vi "Set IConfiguration.vi"(8 "error in":errorcluster, 10 "IConfiguration":refnum<class "IConfiguration.lvclass">, 11 "IVirtual Instrument in":refnum<class "IVirtual Instrument.lvclass">) -> (0 "error out":errorcluster, 3 "IVirtual Instrument out":refnum<class "IVirtual Instrument.lvclass">)   [LabVIEW 2025]
uses:
  IVirtual Instrument.lvclass
  IConfiguration/IConfiguration.lvclass
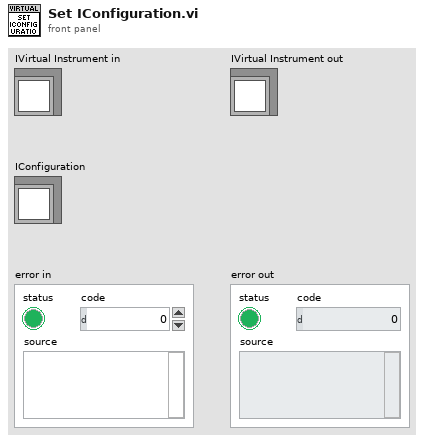
[diagram p1: front panel]
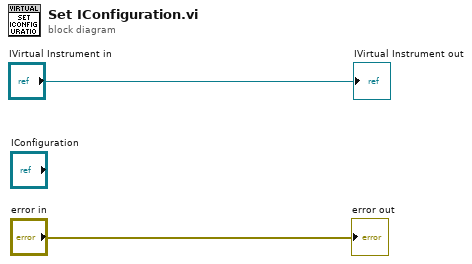
[diagram p0: block diagram]
diagram:
  "IVirtual Instrument out" <- "IVirtual Instrument in"
  "error out" <- "error in"
